vi "Calibration Processing.vi"() -> ()   [LabVIEW 2013]
uses:
  <vilib>/Utility/file.llb/Read From Spreadsheet File (DBL).vi
panel:
  out "Counts/Sec":dbl
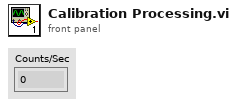
[diagram p1: front panel]
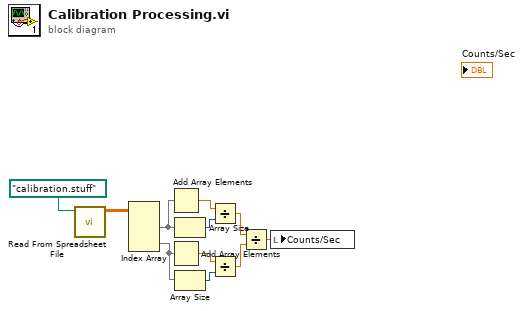
[diagram p0: block diagram]
diagram:
  n1 = call-poly <vilib>:"Read From Spreadsheet File.vi"("file path (dialog if empty)"=path "calibration.stuff" ("new file path (Not A Path if cancelled)")) -> ("all rows"=w10:dbl[][])  [unwired: 6 in, 4 out]
  n2 = Index Array(array=w10) -> (element #1=w9:dbl[], element #2=w4:dbl[])  [unwired: 4 in]
  n3 = Add Array Elements(numeric array=w9) -> (sum=w8:dbl)
  n4 = Add Array Elements(numeric array=w4) -> (sum=w6:dbl)
  n5 = Array Size(array=w9) -> (size(s)=w7:i32)
  n6 = Array Size(array=w4) -> (size(s)=w5:i32)
  n7 = Divide(x=w8, y=w7) -> (x/y=w3:dbl)
  n8 = Divide(x=w6, y=w5) -> (x/y=w2:dbl)
  n9 = Divide(x=w3, y=w2) -> (x/y=w1:dbl)
  n10 = local write "Counts/Sec"(w1) -> ()
